vi "WaitForMoveComplete.vi"(0 "Motion Settings":T1={"No Motion?"=FALSE, "Motion System"=enum."NI 735x", "Motion Bd ID"=1, "Motion Profile"="SMAC1", "# Axis"=1, "Reverse Z axis?"=TRUE, "SMAC Axis"=0, "scan pair"=enum."y-(x) scan", "RT fps"=6.0, "Steps per mm"=[1000, 1000, 1000, 1000], "Motor Parameters"={"velocity ct/s"=[10000.0, 10000.0, 10000.0, 50000.0], "accel ct/s^2"=[50000.0, 50000.0, 50000.0, 200000.0]}, "One Way Scan"=FALSE, "Reverse One Way Scan"=FALSE, "Global Position (mm)"=[], "Plane"=0, "Distance between\nscan lines (um)"=0.0, "Distance between\nscan planes (um)"=0.0, "number of scan planes"=1, "Total steps in line"=0, "Xtra plane\ndistance  (um)"=100, "Xtra planes "=1, "Add Axis"=FALSE, "overshoot cts"=200, "BKPT Shift"=0, "Scan Start Time (ms)"=0, "ESP VISA"="GPIB::1::INSTR", "3rd Axis"=1, "GL Ref Out"=refnum, "Galil Address"=""} {"3rd Axis" items=["x", "y", "z", "w"]; "Xtra planes" min=1; "Xtra plane\ndistance  (um)" min=0; "Distance between\nscan planes (um)" format="%.2f"; "Distance between\nscan lines (um)" format="%.2f"; "SMAC Axis" items=["None"=0, "Axis 1"=1, "Axis 2"=2, "Axis 3"=3, "Axis 4"=4, "Axis 5"=5, "Axis 6"=6, "Axis 7"=7, "Axis 8"=8, "Vector Space 1"=17, "Vector Space 2"=18, "Vector Space 3"=19, "Vector Space 4"=20]; "Motion Bd ID" min=1 max=32 step=1}, 1 "Axis to Ignore (x=1)":i32, 2 "error in":errorcluster, 3 "Ignore Axis?":bool) -> (6 "error out":errorcluster)   [LabVIEW 2022 SP3]
uses:
  MotionParameters.ctl
  MotionSys.ctl
  -MotionRoutines/ScanAxis.ctl
  -MotionRoutines/3rdAxis.ctl
panel:
  # "1-D and 2-D B scan settings"
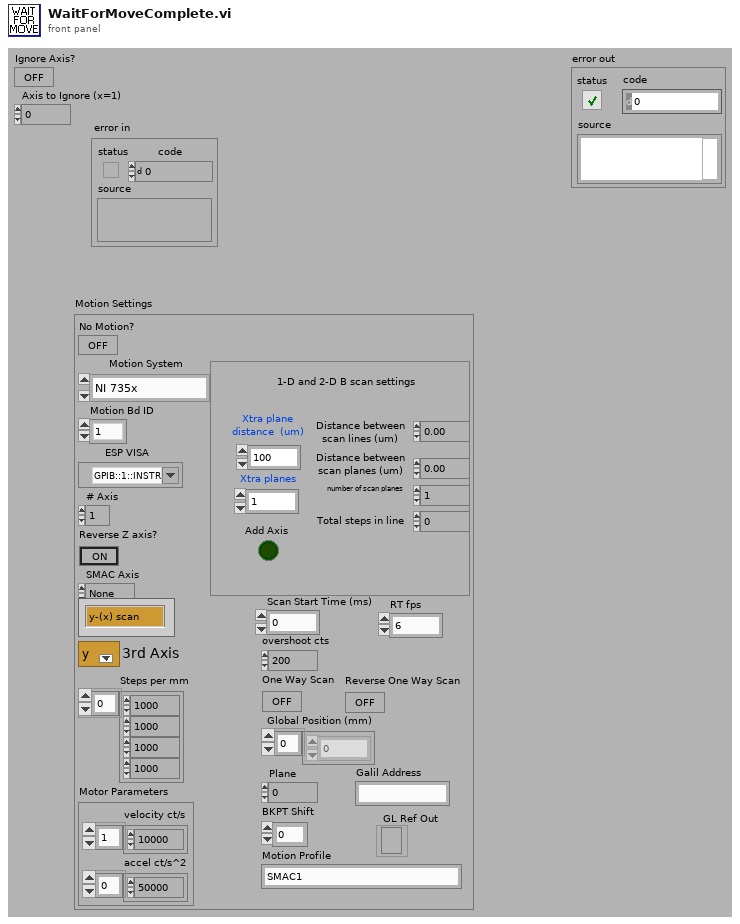
[diagram p1: front panel]
types:
  T1 = typedef "MotionParameters.ctl" = cluster{"No Motion?":bool, "Motion System":T2, "Motion Bd ID":u8, "Motion Profile":string, "# Axis":i8, "Reverse Z axis?":bool, "SMAC Axis":u16, "scan pair":T3, "RT fps":sgl, "Steps per mm":i32[], "Motor Parameters":cluster{"velocity ct/s":dbl[], "accel ct/s^2":dbl[]}, "One Way Scan":bool, "Reverse One Way Scan":bool, "Global Position (mm)":dbl[], "Plane":i32, "Distance between\nscan lines (um)":sgl, "Distance between\nscan planes (um)":sgl, "number of scan planes":i32, "Total steps in line":i32, "Xtra plane\ndistance  (um)":i32, "Xtra planes ":i32, "Add Axis":bool, "overshoot cts":i32, "BKPT Shift":i32, "Scan Start Time (ms)":u32, "ESP VISA":refnum<visa-resource-name>, "3rd Axis":T4, "GL Ref Out":refnum<k7>, "Galil Address":string}
  T2 = typedef "MotionSys.ctl" = enum16{"MM3000", "NI 735x", "Newport ESP", "No Motion Card", "Galil"}
  T3 = typedef "ScanAxis.ctl" = enum16{"y-(x) scan", "x-(y) scan", "z-(x) scan", "z-(y) scan", "y-(z) scan", "x-(z) scan", "w-(x) scan", "w-(y) scan", "w-(z) scan", "x-(w) scan", "y-(w) scan", "z-(w) scan"}
  T4 = typedef "3rdAxis.ctl" = u16
  T5 = cluster{"Reserved":bool, "Axis #1 Move Complete":bool, "Axis #2 Move Complete":bool, "Axis #3 Move Complete":bool, "Axis #4 Move Complete":bool, "Axis #5 Move Complete":bool, "Axis #6 Move Complete":bool, "Axis #7 Move Complete":bool, "Axis #8 Move Complete":bool, "Axis #9 MoveComplete":bool, "Axis #10 Move Complete":bool, "Axis #11 Move Complete":bool, "Axis #12 Move Complete":bool, "Status #13":bool, "Status #14":bool, "Status #15":bool}
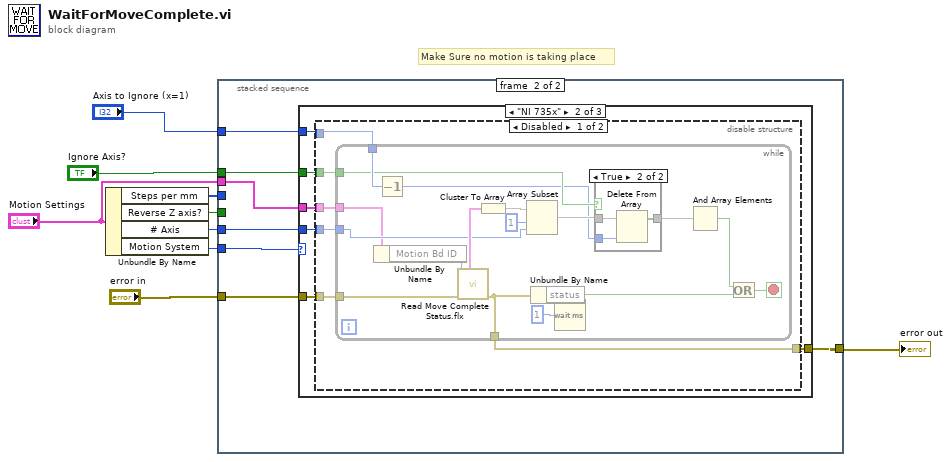
[diagram p0: block diagram]
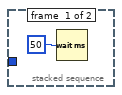
[diagram p2: hidden frame]
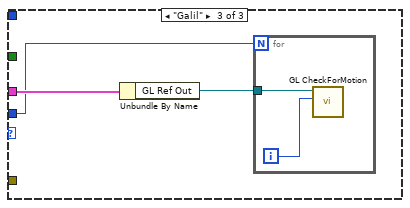
[diagram p6: hidden frame]
diagram:
  # "Make Sure no motion is taking place"
  n1 = Unbundle By Name("Motion Settings") -> ("Steps per mm"=w7:i32[], "Reverse Z axis?"=w6:bool, "# Axis"=w8:i8, "Motion System"=w1:T2)
  n2 = stacked-sequence {
    tunnel: "error in" -> [_ w17]
    tunnel: w8 -> [_ w16]
    tunnel: w7 -> [_ _]
    tunnel: w6 -> [_ _]
    tunnel: "Motion Settings" -> [_ w11]
    tunnel: [_ w15] -> w4
    tunnel: "Axis to Ignore (x=1)" -> [_ w14]
    tunnel: "Ignore Axis?" -> [_ w13]
    tunnel: w1 -> [_ w12]
    frame #0 {
      n3 = Wait (ms)(milliseconds to wait=50) -> ()  [unwired: 1 out]
    }
    frame #1 {
      n4 = case shown="\"NI 735x\"" w12 {
        tunnel: w17 -> [_ w23 _]
        tunnel: w16 -> [_ w22 w51]
        tunnel: [_ w21 _] -> w15
        tunnel: w14 -> [_ w20 _]
        tunnel: w13 -> [_ w19 _]
        tunnel: w11 -> [_ w18 w53]
        frame "MM3000", Default {
        }
        frame "NI 735x" {
          n5 = disable-structure shown="Disabled" {
            disable-tunnel: w23 -> [w29 _]
            disable-tunnel: w22 -> [w28 _]
            disable-tunnel: [w27 _] -> w21
            disable-tunnel: w20 -> [w26 _]
            disable-tunnel: w19 -> [w25 _]
            disable-tunnel: w18 -> [w24 _]
            frame Disabled {
              n6 = while {
                tunnel: w29 -> [w43]
                tunnel: w28 -> [w40]
                tunnel: [w42] -> w27
                tunnel: w26 -> [w37]
                tunnel: w25 -> [w36]
                tunnel: w24 -> [w31]
                stop <- w45 stop-if-true
                n7 = Unbundle By Name(w31) -> ("Motion Bd ID"=w30:u8)
                n8 = Decrement(x=w37) -> (x-1=w32:i32)
                n9 = call <vilib>:"Read Move Complete Status.flx"("error in (no error)"=w43, "Board ID"=w30) -> ("error out"=w42:errorcluster, "Move Complete Status"=w46:T5)  [unwired: 1 in, 4 out]
                n10 = Cluster To Array(cluster=w46) -> (array=w35:bool[])
                n11 = Array Subset(array=w35, index=1, length=w40) -> (w33:bool[])
                n12 = Unbundle By Name(w42) -> ("status"=w38:bool)
                n13 = Wait (ms)(milliseconds to wait=1) -> ()  [unwired: 1 out]
                n14 = case shown="True" w36 {
                  tunnel: w33 -> [w47 w50]
                  tunnel: w32 -> [_ w49]
                  tunnel: [w47 w48] -> w34
                  frame False {
                  }
                  frame True {
                    n15 = Delete From Array(array=w50, index=w49) -> (array with subset deleted=w48:bool[])  [unwired: 1 in, 1 out]
                  }
                }
                n16 = And Array Elements(Boolean array=w34) -> (logical AND=w39:bool)
                n17 = Or(x=w39, y=w38) -> (x .or. y?=w45:bool)
              }
            }
            frame Enabled {
            }
          }
        }
        frame "Galil" {
          n18 = Unbundle By Name(w53) -> ("GL Ref Out"=w52:refnum<k7>)
          n19 = for {
            N: w51 -> [_]
            tunnel: w52 -> [w55]
            i -> [w54]
            n20 = call "GL CheckForMotion.vi"("Axis"=w54, "Refnum in"=w55) -> ()  [unwired: 7 in, 3 out]
          }
        }
      }
    }
  }
  "error out" <- w4
